vi "HostTest.vi"() -> ()   [LabVIEW 2017]
uses:
  <vilib>/NI/PowerElectronicsControl/ScaleAndLimit/Interface/Configuration.ctl
  <instrlib>/_niInstr/FIFO Register Bus/v1/Host/niInstr FIFO Register Bus v1 Host.lvclass
  C:/Program Files (x86)/National Instruments/LabVIEW 2017/instr.lib/_niInstr/Instruction Framework/v1/Host/Instruction Target/niInstr Instruction Target v1 Host.lvclass
  <vilib>/FPGAPlugInAG/sbRIO-9607/niLvFpga_Open_sbRIO-9607.vi
  <vilib>/rvi/interface/common/dynamic/niFpgaDynamicAddResources.vi
  <vilib>/FPGAPlugInAG/Dynamic/niLvFpga_Reset_Dynamic.vi
  <vilib>/Utility/error.llb/Error Cluster From Error Code.vi
  <vilib>/rvi/errors/niLvFpgaAdjustHostInterfaceError.vi
  <vilib>/FPGAPlugInAG/Dynamic/niLvFpga_Run_Dynamic.vi
  <vilib>/NI/PowerElectronicsControl/WaveformAcq/RT/ReadWaveform.vi
  <vilib>/FPGAPlugInAG/Dynamic/niLvFpga_Close_Dynamic.vi
  <vilib>/rvi/interface/nirviOpenFPGA/nirviOpenFPGA.xnode
  FPGA Bitfiles/AFE_FPGATarget_CoreTestHarness_+BccrjhzUL4.lvbitx
  CoreTestHarness.vi
  <vilib>/rvi/interface/nirviMethod/nirviMethod.xnode
  <vilib>/rvi/interface/nirviReadWriteControl/nirviReadWriteControl.xnode
  <vilib>/rvi/interface/nirviCloseFPGA/nirviCloseFPGA.xnode
  <vilib>/NI/PowerElectronicsControl/WaveformAcq/RT/WaveformTask.lvclass
  <vilib>/NI/PowerElectronicsControl/ScaleAndLimit/Interface/ScaleAndLimitInterface.lvlib
  <instrlib>/_niInstr/Instruction Framework/v1/Host/Subsystem Map/niInstr Subsystem Map v1 Host.lvclass
  NiFpgaLv.dll
  <vilib>/rvi/interface/Simulation/niFpgaSimulationCallBeginRW.vi
  <vilib>/NI/PowerElectronicsControl/SVPWM/SVPWMInterface/SVPWMInterface.lvlib
panel:
  in  "Tabs":T1(tab)
  in  "AFE_ControlSignals":cluster{"resetPLL":bool, "resetControl":bool}
  in  "UpdateAFE":bool
  in  "AFE_Setpoints":cluster{"VDCLink":sgl, "DirectedIdSetpt":sgl}
  in  "AFE_ManualControl":T2
  in  "AFE_Gains":T3
  out "actualAFErate":i16
  out "Limits":string
  out "SimultaneousAILoopRate":u32
  in  "clearLimits":bool
  in  "stop":bool
  out "Data":waveform(sgl)[](graph)
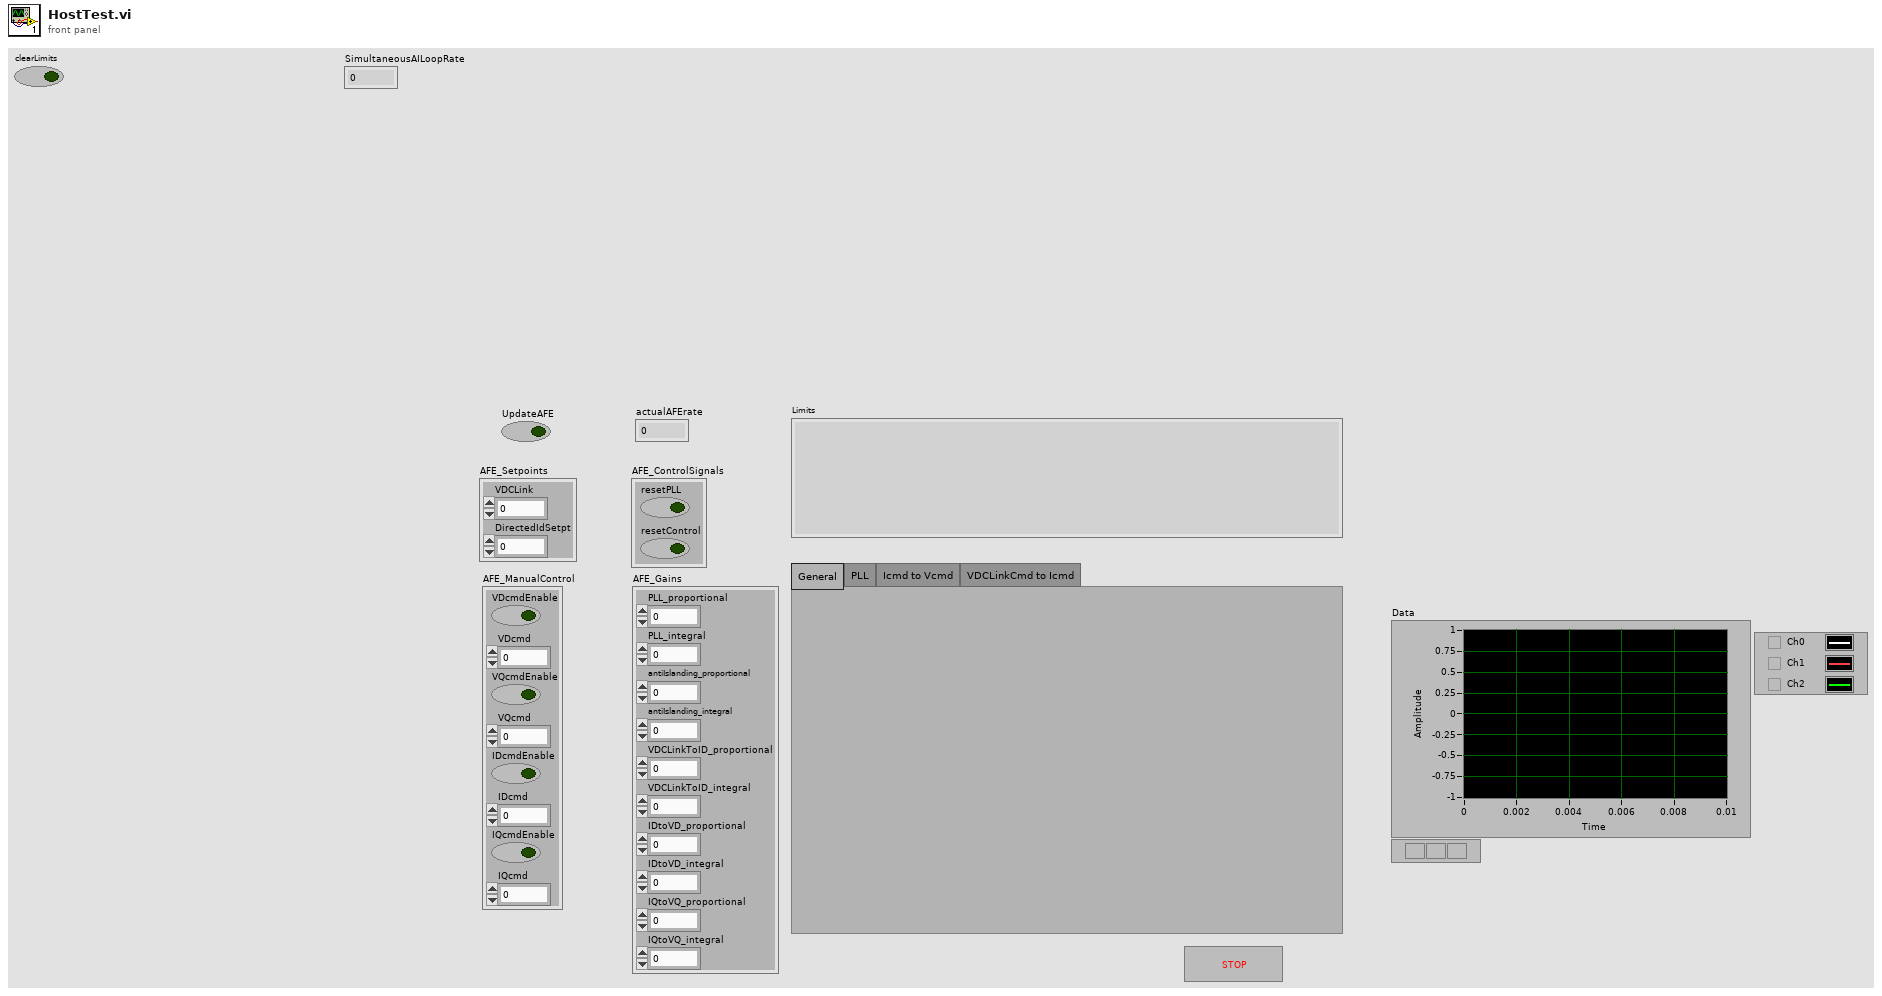
[diagram p1: front panel]
types:
  T1 = enum32{"General", "PLL", "Icmd to Vcmd", "VDCLinkCmd to Icmd"}
  T2 = cluster{"VDcmdEnable":bool, "VDcmd":sgl, "VQcmdEnable":bool, "VQcmd":sgl, "IDcmdEnable":bool, "IDcmd":sgl, "IQcmdEnable":bool, "IQcmd":sgl}
  T3 = cluster{"PLL_proportional":sgl, "PLL_integral":sgl, "antiIslanding_proportional":sgl, "antiIslanding_integral":sgl, "VDCLinkToID_proportional":sgl, "VDCLinkToID_integral":sgl, "IDtoVD_proportional":sgl, "IDtoVD_integral":sgl, "IQtoVQ_proportional":sgl, "IQtoVQ_integral":sgl}
  T4 = cluster{"PLL_PIRad_high":sgl, "PLL_PiRad_low":sgl, "IQcmd_high":sgl, "IQcmd_low":sgl, "IDcmd_high":sgl, "IDcmd_low":sgl, "VDcmd_high":sgl, "VDcmd_low":sgl, "VQmcd_high":sgl, "VQcmd_low":sgl}
  T5 = typedef "ScaleAndLimitInterface.lvlib/Configuration.ctl" = cluster{"Name":string, "M":dbl, "B":i16, "HighLimit":dbl, "LowLimit":dbl, "LimitsEnabled":bool}
  T6 = typedef "SVPWMInterface.lvlib/Configuration.ctl" = cluster{"Deadtime":u8, "Period":u32}
  T7 = typedef "ScaleAndLimitInterface.lvlib/Interface.ctl" = cluster{"instruction target":refnum<class "niInstr Instruction Target v1 Host.lvclass">, "ScalingAndLimitsContext":refnum<class "niInstr Instruction Framework Context v1 Host.lvclass">, "Configuration":T5[]}
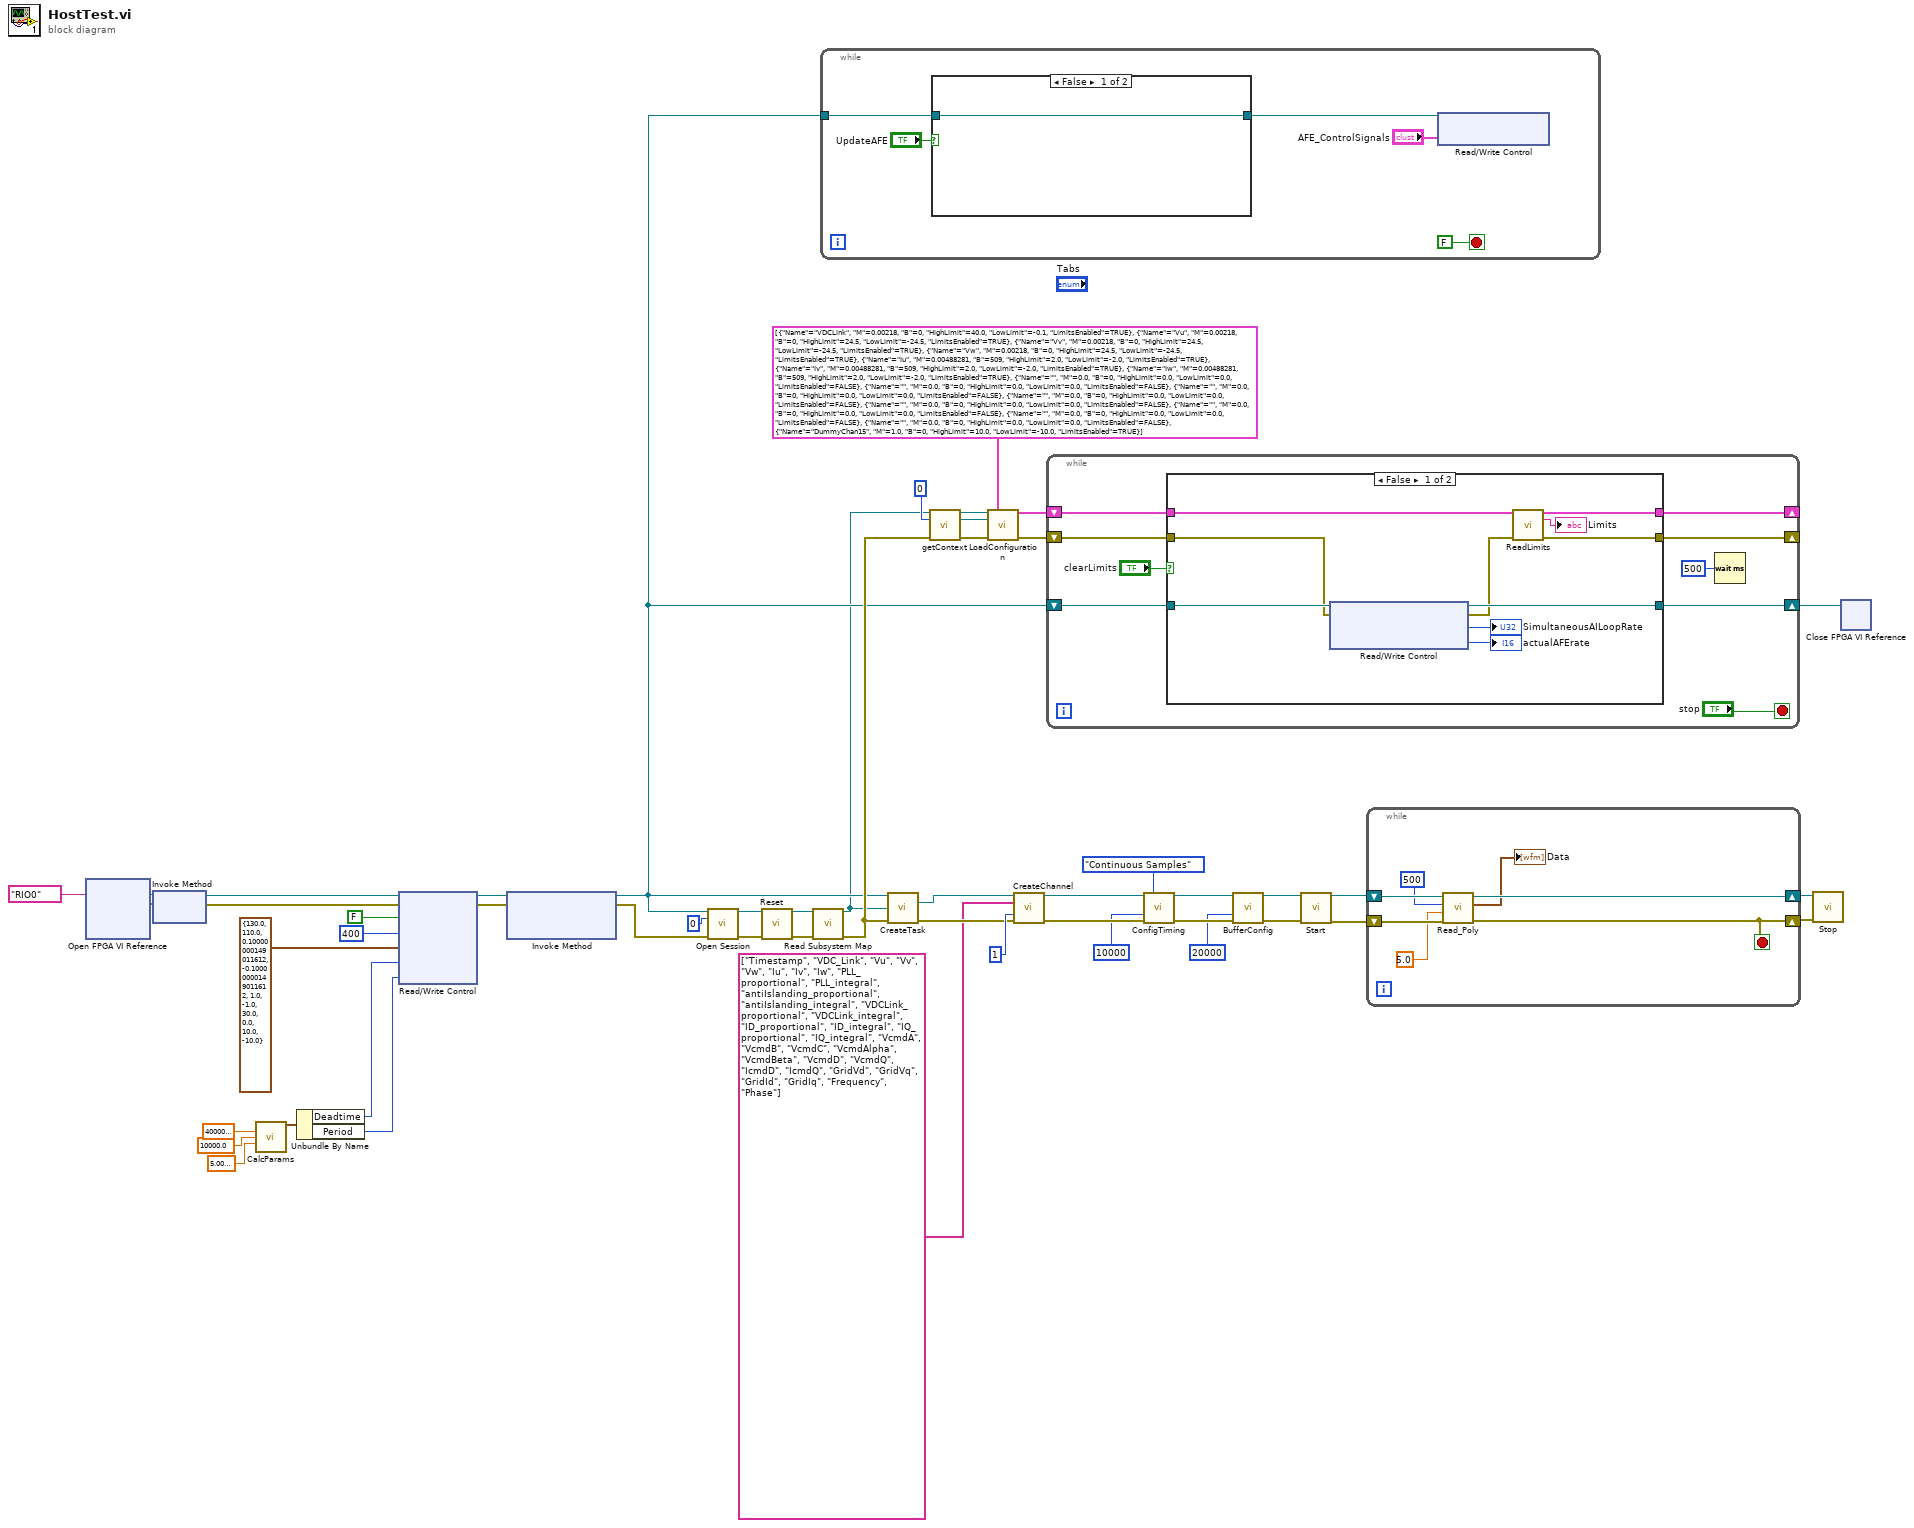
[diagram p0: block diagram]
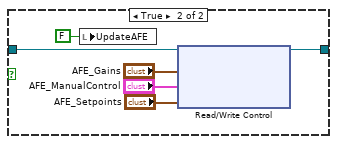
[diagram p2: hidden frame]
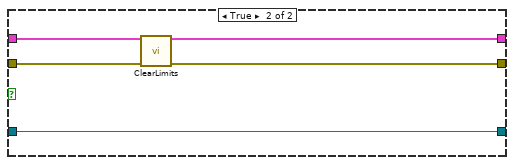
[diagram p3: hidden frame]
diagram:
  n1 = xnode "Open FPGA VI Reference"("resource name"=tag "RIO0") -> ("FPGA VI Reference Out"=w29:refnum<k20>, "error out"=w28:errorcluster)  [unwired: 1 in]
  n2 = xnode "Invoke Method"("FPGA VI Reference In"=w29, "error in"=w28) -> ("FPGA VI Reference Out"=w15:refnum<k20>, "error out"=w14:errorcluster)
  n3 = call <vilib>:"CalcParams.vi"("ClkRate"=sgl 40000000.0, "fc"=sgl 10000.0, "deadtime"=sgl 5e-08) -> ("Configuration"=w5:T6)  [unwired: 12 in]
  n4 = Unbundle By Name(w5) -> ("Deadtime"=w4:u8, "Period"=w3:u32)
  n5 = xnode "Read/Write Control"("FPGA VI Reference In"=w15, "error in"=w14, "enableIGBTs"=FALSE, "AFE_rate"=i16 400, "AFE_Range"=T4 {"PLL_PIRad_high"=130.0, "PLL_PiRad_low"=110.0, "IQcmd_high"=0.1, "IQcmd_low"=-0.1, "IDcmd_high"=1.0, "IDcmd_low"=-1.0, "VDcmd_high"=30.0, "VDcmd_low"=0.0, "VQmcd_high"=10.0, "VQcmd_low"=-10.0}, "Deadtime"=w4, "Period"=w3) -> ("FPGA VI Reference Out"=w13:refnum<k20>, "error out"=w12:errorcluster)
  n6 = xnode "Invoke Method"("FPGA VI Reference In"=w13, "error in"=w12) -> ("FPGA VI Reference Out"=w2:refnum<k20>, "error out"=w31:errorcluster)  [unwired: 1 in]
  n7 = call <instrlib>:"Open Session.vi"("fpga ref"=w2, "bus instance"=u32 0, "error in"=w31) -> ("session out"=w33:refnum<class "niInstr FIFO Register Bus v1 Host.lvclass">, "error out"=w34:errorcluster)  [unwired: 11 in]
  n8 = call-dynamic "Reset.vi"("session in"=w33, "error in"=w34) -> ("session out"=w18:refnum<class "niInstr FIFO Register Bus v1 Host.lvclass">, "error out"=w17:errorcluster)  [unwired: 12 in]
  n9 = call <instrlib>:"Read Subsystem Map.vi"("instruction target in"=w18, "error in"=w17) -> ("instruction target out"=w1:refnum<class "niInstr FIFO Register Bus v1 Host.lvclass">, "error out"=w16:errorcluster)  [unwired: 11 in, 1 out]
  n10 = while {
    tunnel: w2 -> [w54]
    stop <- FALSE stop-if-true
    n11 = case shown="False" "UpdateAFE" {
      tunnel: w54 -> [w56 w62]
      tunnel: [w56 w58] -> w52
      frame False {
      }
      frame True {
        n12 = local write "UpdateAFE"(FALSE ("UpdateAFE")) -> ()
        n13 = xnode "Read/Write Control"("FPGA VI Reference In"=w62, "AFE_Gains"="AFE_Gains", "AFE_ManualControl"="AFE_ManualControl", "AFE_Setpoints"="AFE_Setpoints") -> ("FPGA VI Reference Out"=w58:refnum<k20>)  [unwired: 1 in, 1 out]
      }
    }
    n14 = xnode "Read/Write Control"("FPGA VI Reference In"=w52, "AFE_ControlSignals"="AFE_ControlSignals") -> ()  [unwired: 1 in, 2 out]
  }
  n15 = call <vilib>:"CreateTask.vi"("FPGA Ref in"=w2, "session in"=w1, "error in"=w16) -> ("Task out"=w38:refnum<class "WaveformTask.lvclass">, "error out"=w37:errorcluster)  [unwired: 9 in, 2 out]
  n16 = call <vilib>:"getContext.vi"("session in"=w1, "instance"=u8 0, "error in"=w16) -> ("session out"=w20:refnum<class "niInstr FIFO Register Bus v1 Host.lvclass">, "ScalingAndLimitsContext"=w19:refnum<class "niInstr Instruction Framework Context v1 Host.lvclass">, "error out"=w26:errorcluster)  [unwired: 10 in]
  n17 = call <vilib>:"LoadConfiguration.vi"("instruction target in"=w20, "Configuration"=T5[] [{"Name"="VDCLink", "M"=0.00218, "B"=0, "HighLimit"=40.0, "LowLimit"=-0.1, "LimitsEnabled"=TRUE}, {"Name"="Vu", "M"=0.00218, "B"=0, "HighLimit"=24.5, "LowLimit"=-24.5, "LimitsEnabled"=TRUE}, {"Name"="Vv", "M"=0.00218, "B"=0, "HighLimit"=24.5, "LowLimit"=-24.5, "LimitsEnabled"=TRUE}, {"Name"="Vw", "M"=0.00218, "B"=0, "HighLimit"=24.5, "LowLimit"=-24.5, "LimitsEnabled"=TRUE}, {"Name"="Iu", "M"=0.00488281, "B"=509, "HighLimit"=2.0, "LowLimit"=-2.0, "LimitsEnabled"=TRUE}, {"Name"="Iv", "M"=0.00488281, "B"=509, "HighLimit"=2.0, "LowLimit"=-2.0, "LimitsEnabled"=TRUE}, {"Name"="Iw", "M"=0.00488281, "B"=509, "HighLimit"=2.0, "LowLimit"=-2.0, "LimitsEnabled"=TRUE}, {"Name"="", "M"=0.0, "B"=0, "HighLimit"=0.0, "LowLimit"=0.0, "LimitsEnabled"=FALSE}, {"Name"="", "M"=0.0, "B"=0, "HighLimit"=0.0, "LowLimit"=0.0, "LimitsEnabled"=FALSE}, {"Name"="", "M"=0.0, "B"=0, "HighLimit"=0.0, "LowLimit"=0.0, "LimitsEnabled"=FALSE}, {"Name"="", "M"=0.0, "B"=0, "HighLimit"=0.0, "LowLimit"=0.0, "LimitsEnabled"=FALSE}, {"Name"="", "M"=0.0, "B"=0, "HighLimit"=0.0, "LowLimit"=0.0, "LimitsEnabled"=FALSE}, {"Name"="", "M"=0.0, "B"=0, "HighLimit"=0.0, "LowLimit"=0.0, "LimitsEnabled"=FALSE}, {"Name"="", "M"=0.0, "B"=0, "HighLimit"=0.0, "LowLimit"=0.0, "LimitsEnabled"=FALSE}, {"Name"="", "M"=0.0, "B"=0, "HighLimit"=0.0, "LowLimit"=0.0, "LimitsEnabled"=FALSE}, {"Name"="DummyChan15", "M"=1.0, "B"=0, "HighLimit"=10.0, "LowLimit"=-10.0, "LimitsEnabled"=TRUE}], "ScalingAndLimitsContext"=w19, "error in (no error)"=w26) -> ("Interface"=w23:T7, "error out"=w22:errorcluster)  [unwired: 10 in]
  n18 = call <vilib>:"CreateChannel.vi"("task in"=w38, "Chan Name Array"=string[] ["Timestamp", "VDC_Link", "Vu", "Vv", "Vw", "Iu", "Iv", "Iw", "PLL_proportional", "PLL_integral", "antiIslanding_proportional", "antiIslanding_integral", "VDCLink_proportional", "VDCLink_integral", "ID_proportional", "ID_integral", "IQ_proportional", "IQ_integral", "VcmdA", "VcmdB", "VcmdC", "VcmdAlpha", "VcmdBeta", "VcmdD", "VcmdQ", "IcmdD", "IcmdQ", "GridVd", "GridVq", "GridId", "GridIq", "Frequency", "Phase"], "instance"=u8 1, "error in"=w37) -> ("Task out"=w39:refnum<class "WaveformTask.lvclass">, "error out"=w49:errorcluster)  [unwired: 10 in]
  n19 = while {
    shift-right: [w65] -> _
    shift-left: w23 -> [w71]
    shift-right: [w64] -> _
    shift-left: w22 -> [w70]
    shift-right: [w66] -> w21
    shift-left: w2 -> [w67]
    stop <- "stop" stop-if-true
    n20 = case shown="False" "clearLimits" {
      tunnel: w71 -> [w78 w86]
      tunnel: w70 -> [w80 w85]
      tunnel: [w77 w84] -> w65
      tunnel: [w76 w83] -> w64
      tunnel: w67 -> [w81 w82]
      tunnel: [w79 w82] -> w66
      frame False {
        n21 = xnode "Read/Write Control"("FPGA VI Reference In"=w81, "error in"=w80) -> ("FPGA VI Reference Out"=w79:refnum<k20>, "error out"=w74:errorcluster, "SimultaneousAILoopRate"=→"SimultaneousAILoopRate":u32, "actualAFErate"=→"actualAFErate":i16)
        n22 = call <vilib>:"ReadLimits.vi"("Interface in"=w78, "error in (no error)"=w74) -> ("Interface out"=w77:T7, "Limits"=→"Limits":string, "error out"=w76:errorcluster)  [unwired: 11 in]
      }
      frame True {
        n23 = call <vilib>:"ClearLimits.vi"("Interface in"=w86, "error in (no error)"=w85) -> ("Interface out"=w84:T7, "error out"=w83:errorcluster)  [unwired: 12 in]
      }
    }
    n24 = Wait (ms)(milliseconds to wait=u32 500) -> ()  [unwired: 1 out]
  }
  n25 = call <vilib>:"ConfigTiming.vi"("Task in"=w39, "Sample Mode"=enum16{"Finite Samples", "Continuous Samples"}."Continuous Samples", "Sample Rate"=u32 10000, "error in (no error)"=w49) -> ("Task out"=w46:refnum<class "WaveformTask.lvclass">, "error out"=w45:errorcluster)  [unwired: 9 in, 1 out]
  n26 = call <vilib>:"BufferConfig.vi"("WaveformTask in"=w46, "Buffer Size [Samps per Chan]"=20000, "error in (no error)"=w45) -> ("WaveformTask out"=w43:refnum<class "WaveformTask.lvclass">, "error out"=w42:errorcluster)  [unwired: 10 in, 1 out]
  n27 = call <vilib>:"Start.vi"("WaveformTask in"=w43, "error in (no error)"=w42) -> ("WaveformTask out"=w41:refnum<class "WaveformTask.lvclass">, "error out"=w40:errorcluster)  [unwired: 12 in]
  n28 = while {
    shift-right: [w87] -> w35
    shift-left: w40 -> [w92]
    shift-right: [w89] -> w36
    shift-left: w41 -> [w93]
    stop <- w87 stop-if-true
    n29 = call-poly <vilib>:"Read_Poly.vi"("error in"=w92, "Timeout (s)"=5.0, "Samps Read per Chan"=500, "Task in"=w93) -> ("error out"=w87:errorcluster, "Waveforms"=→"Data":waveform(sgl)[], "Task out"=w89:refnum<class "WaveformTask.lvclass">)  [unwired: 4 in, 1 out]
  }
  n30 = call <vilib>:"Stop.vi"("error in"=w35, "WaveformTask in"=w36) -> ()  [unwired: 8 in, 2 out]
  n31 = xnode "Close FPGA VI Reference"("FPGA VI Reference In"=w21) -> ()  [unwired: 1 in, 1 out]
